vi "SubVI_Calcular_theta2_a_partir_de_theta3.vi"(1 "theta2 (Graus)":dbl, 2 "theta3 (graus)":dbl) -> (0 "Ângulo":dbl)   [LabVIEW 2017]
panel:
  out "Angulo 2":dbl
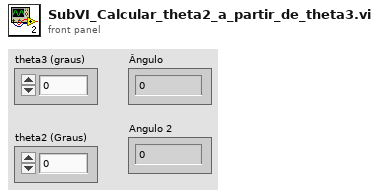
[diagram p1: front panel]
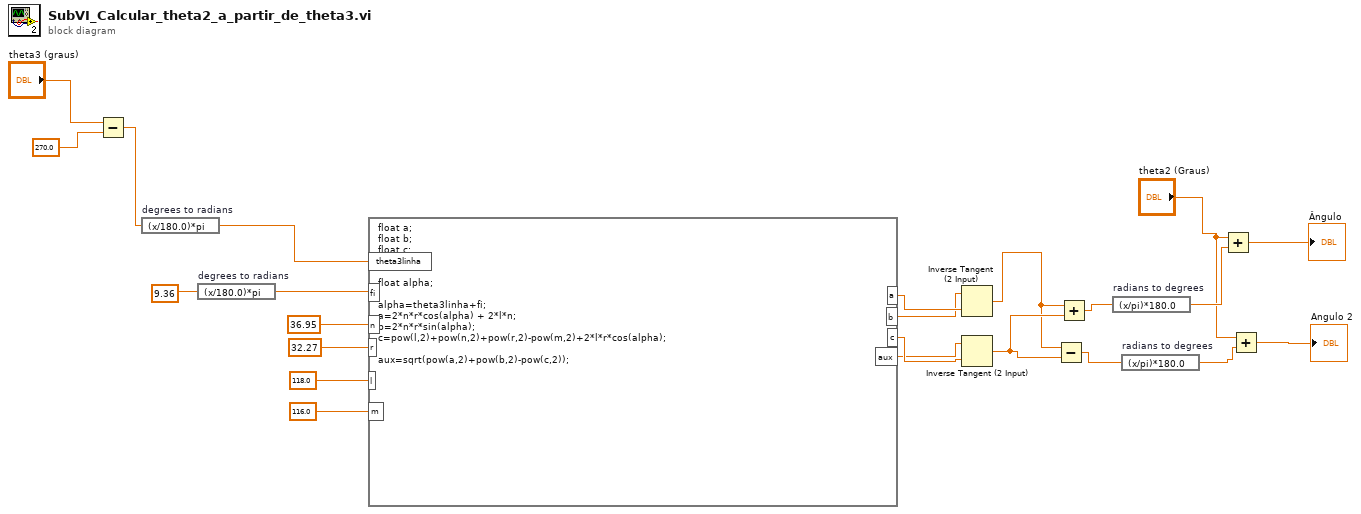
[diagram p0: block diagram]
diagram:
  n1 = Subtract(x="theta3 (graus)", y=270.0) -> (x-y=w8:dbl)
  n2 = expression code="(x/180.0)*pi" "degrees to radians"(w8) -> (w15:dbl)
  n3 = expression code="(x/180.0)*pi" "degrees to radians"(9.36 ("input variable")) -> (w17:dbl)
  n4 = formula code="float a;\nfloat b;\nfloat c;\nfloat aux;\n\nfloat alpha;\n\nalpha=theta3linha+fi;\na=2*n*r*cos(alpha) + 2*l*n;\nb=2*n*r*sin(alpha);\nc=pow(l,2)+pow(n,2)+pow(r,2)-pow(m,2)+2*l*r*cos(alpha);\n\naux=sqrt(pow(a,2)+pow(b,2)-pow(c,2));"("theta3linha"=w15, "fi"=w17, "n"=36.95 ("input variable"), "r"=32.27 ("input variable"), "l"=118.0 ("input variable"), "m"=116.0 ("input variable")) -> ("a"=w14:dbl, "b"=w13:dbl, "c"=w19:dbl, "aux"=w18:dbl)
  n5 = Inverse Tangent (2 Input)(1:w14, 2:w13) -> (0:w20:dbl)
  n6 = Inverse Tangent (2 Input)(1:w19, 2:w18) -> (0:w21:dbl)
  n7 = Subtract(x=w20, y=w21) -> (x-y=w23:dbl)
  n8 = Add(x=w20, y=w21) -> (x+y=w22:dbl)
  n9 = expression code="(x/pi)*180.0" "radians to degrees"(w22) -> (w6:dbl)
  n10 = expression code="(x/pi)*180.0" "radians to degrees"(w23) -> (w4:dbl)
  n11 = Add(x="theta2 (Graus)", y=w6) -> (x+y=→"Ângulo":dbl)
  n12 = Add(x="theta2 (Graus)", y=w4) -> (x+y=→"Angulo 2":dbl)
